vi "Dashboard Main.vi"() -> ()   [LabVIEW 2016]
uses:
  <vilib>/Utility/miscctls.llb/LVRowAndColumnTypeDef.ctl
  <vilib>/event_ctls.llb/eventvkey.ctl
  <vilib>/Rock Robotics/Network Tables/NT Read Boolean.vi
  <vilib>/Rock Robotics/Network Tables/NT Write Boolean.vi
  <vilib>/Rock Robotics/WPI/Dashboard/WPI_DashboardLogging Global.vi
panel:
  in  "Camera Settings Right":T1={"Frame Rate"=30, "Compression"=30, "Size"=1, "DB Camera Config"=FALSE} {"Frame Rate" scale=1.0..30.0; "Compression" scale=100.0..-1.0; "Size" items=["640x480", "320x240", "160x120"]}
  in  "Camera Name Right":string(combo)="No Camera Selection"
  out "Camera Info":cluster{"Mbps LED":bool, "Mbps":dbl, "fps":dbl} {"fps" format="%#.1g"; "Mbps" format="%#.1g"}
  in  "Camera Settings":T1={"Frame Rate"=30, "Compression"=30, "Size"=1, "DB Camera Config"=FALSE} {"Frame Rate" scale=1.0..30.0; "Compression" scale=100.0..-1.0; "Size" items=["640x480", "320x240", "160x120"]}
  in  "TCP":refnum<k5>
  in  "Rec Mode":enum32{"Stop", "Record", "Playback"}(radio)
  out "Robot IP":string
  out "Image Message":string="Timeout in Camera Communications"
  in  "Dashboard Tab":T2(tab)
  in  "Select Auto":string(combo)="Select Autonomous ..."
  out "NT Connection":bool
  out "JS1 Z":dbl(slide) scale=-1.0..1.0 scale format="%#_2e"
  out "JS1 Graph":cluster{"X":dbl, "Y":dbl}[](graph)
  out "JS1 Buttons":T3
  out "JS2 Z":dbl(slide) scale=-1.0..1.0 scale format="%#_2e"
  out "JS2 Graph":cluster{"X":dbl, "Y":dbl}[](graph)
  out "JS2 Buttons":T3
  out "Mode":T4(ring)=enum."Auto Disabled"
  out "Camera Image Right":T5(plugin-control)
  in  "DB/String 9":string
  in  "DB/String 8":string
  in  "DB/String 7":string
  in  "DB/String 6":string
  in  "DB/String 5":string
  in  "DB/String 4":string
  in  "DB/String 3":string
  in  "DB/String 2":string
  in  "DB/String 1":string
  in  "DB/String 0":string
  in  "DB/Slider 0":dbl(slide) scale=0.0..5.0
  in  "DB/Slider 1":dbl(slide) scale=0.0..5.0
  in  "DB/Slider 2":dbl(slide) scale=0.0..5.0
  in  "DB/Slider 3":dbl(slide) scale=0.0..5.0
  out "DB/LED 3":bool
  out "DB/LED 2":bool
  out "DB/LED 1":bool
  out "DB/LED 0":bool
  in  "DB/Button 3":bool
  in  "DB/Button 2":bool
  in  "DB/Button 1":bool
  in  "DB/Button 0":bool caption="New Name"
  in  "Station3":bool
  in  "Station2":bool
  in  "Station1":bool
  in  "ClimberSpeed":dbl(slide)=0.9067796610169492 scale=0.0..1.0
  out "Commanded Angle":dbl
  out "Sonar-Inches":dbl
  out "Encoder-Inches":dbl
  out "Gyro-Degrees":dbl
  out "Battery V":dbl
  out "Doors":bool
  out "Compressor":bool
  in  "Min Area Size %":dbl=20.0
  in  "Lower Threshold":dbl=50.0
  out "Hook Center":dbl
  in  "Test Slider":dbl(slide) scale=0.0..100.0 scale format="%#_3g"
  in  "On/Off":bool caption="Solenoid"
  in  "Test Name":u16(ring) items=["Select the test to run..."]
  in  "Test Tree":string(tree)
  in  "Motor":cluster{"Value":dbl, "Enable":bool} {"Value" scale=-1.0..1.0 scale format="%#_3g"}
  out "Progress":T6 {"Test Progress" scale=0.0..100.0}
  in  "Rev/Fwd":cluster{"Forward":bool, "Reverse":bool}
  in  "Test Ring":u16(ring) items=["Monochrome", "Color"]
  out "Cmd Status":string
  in  "Execute Command":bool
  in  "Command Params":string[][](table)
  in  "Command Selection":i32(listbox)
  in  "CheckList":i32(listbox)
  out "Tree":string(tree)
  out "Camera Image":T5(plugin-control)
  out "Background":bool
  in  "Camera Name":string(combo)="No Camera Selection"
  # "HW"
  # "HW"
  # "Joysticks"
  # "Drive Motors"
  # "Front"
  # "Right"
  # "Left"
  # "Back"
  # "Closed"
  # "Open"
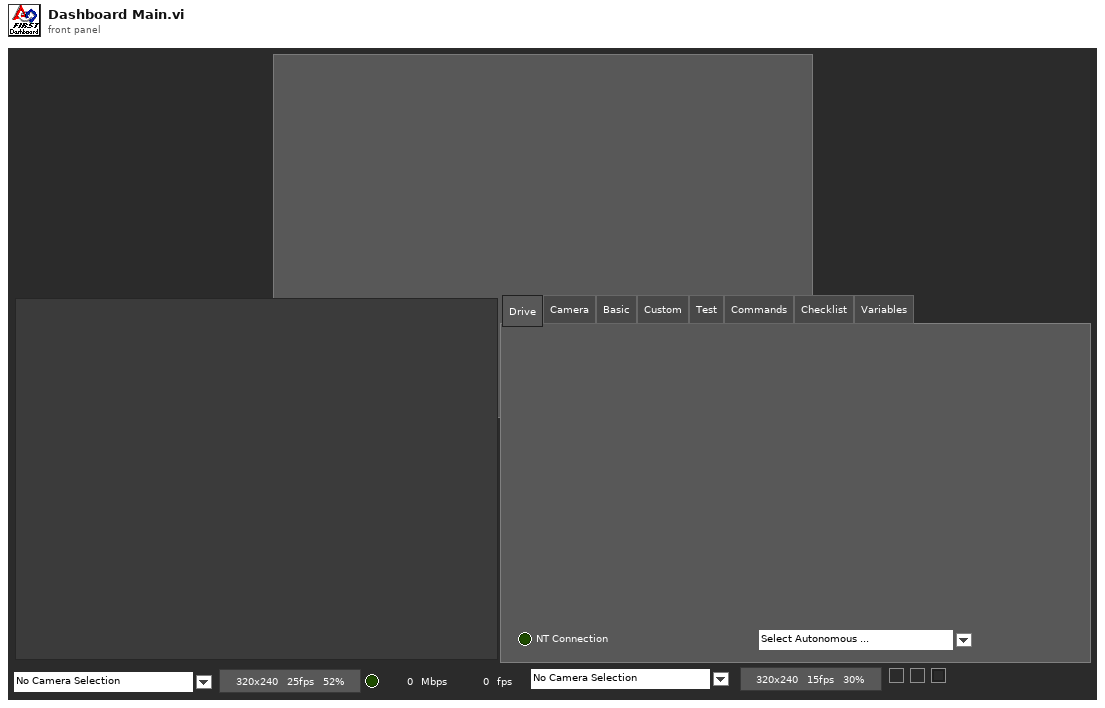
[diagram p1: front panel]
types:
  T1 = cluster{"Frame Rate":i32, "Compression":i32, "Size":u16, "DB Camera Config":bool}
  T2 = enum32{"Drive", "Camera", "Basic", "Custom", "Test", "Commands", "Checklist", "Variables"}
  T3 = cluster{bool, bool, bool, bool, bool, bool, bool, bool, bool, bool, bool, bool}
  T4 = enum8{"Tele-Op Disabled", "Tele-Op Enabled", "Auto Disabled", "Auto Enabled", "Test Disabled", "Test Enabled", "Disconnected", "No Code", "E-Stop"}
  T5 = typedef "IMAQ Image.ctl" = refnum<image>
  T6 = cluster{"Test Progress":u8, "Test Progress Text":string}
  T7 = typedef "Image Type" = u32
  T8 = cluster{"IDs":cluster{"RPC field ID":u16, "Unique ID":u16}, "String":string}
  T9 = enum32{"Drive", "Basic", "Custom", "Test", "Checklist", "Variables"}
  T10 = cluster{"Camera Image":refnum<vi>, "Dashboard Tab":refnum<vi>, "Background":refnum<vi>, "Rec Mode":refnum<vi>, "Test Slider":refnum<vi>, "On/Off ":refnum<vi>, "Test Ring":refnum<vi>, "Rev/Fwd":refnum<vi>, "Test Name":refnum<vi>, "Motor":refnum<vi>, "Progress":refnum<vi>, "CheckList":refnum<vi>, "Tree":refnum<vi>, "Test Tree":refnum<vi>, "Command Params":refnum<vi>, "Command Selection":refnum<vi>, "Execute Command":refnum<vi>, "Cmd Status":refnum<vi>, "Camera Settings":refnum<vi>, "Camera Name":refnum<vi>, "Camera Info":refnum<vi>, "Camera Settings Right":refnum<vi>, "Camera Name Right":refnum<vi>, "Camera Image Right":refnum<vi>}
  T11 = cluster{"Error Strings":string, "Disable Counts":cluster{u16, u16}, "Rail Faults":cluster{u16, u16, u16}, "Robot IP":string, "DB Mode":u8, "Event Info":cluster{"Name":string, "Type":u8, "Number":u16, "Replay":u8}}
  T12 = cluster{"Storage":cluster{"Disk Free":u64, "RAM Block":u32, "RAM free":u32}, "CPU Utilization":cluster{"CPU % ISR":sgl, "CPU % Time Crit":sgl, "CPU % Timed Str":sgl, "CPU % High":sgl, "CPU % Above":sgl, "CPU % Normal":sgl, "CPU % Low":sgl}, "CAN":cluster{"% Bus Utilization":sgl, "Bus Off Cnt":u32, "TX_FIFO Full Cnt":u32, "Receive Error Cnt":u8, "Transmit Error Cnt":u8}, "HID":cluster{"HID Outputs":u32, "Rumble Low":u16, "Rumble High":u16}[]}
  T13 = cluster{"Status bits":cluster{"Test Mode":bool, "Autonomous":bool, "Enabled":bool, "Code Start":bool, "Brownout":bool, "Reserved 2":bool, "Reserved 3":bool, "E-Stop":bool}, "Code Trace":cluster{"Disabled":bool, "TeleOp":bool, "Auto":bool, "Test":bool}, "Controller Type":enum16{"unknown", "cRIO", "roboRio"}, "Code?":enum16{"unknown", "noCode", "code"}, "Battery V":dbl}
  T14 = cluster{"Control Bits":cluster{"TestMode":bool, "Autonomous":bool, "Enabled":bool, "FMS Present":bool, bool, bool, bool, "E-Stop":bool}, "Team Station ":u8, "Countdown":sgl, "Joystick Values":cluster{"Axes":dbl[], "Buttons":bool[], "POVs":i16[]}[]}
  T15 = cluster{"Axes":dbl[], "Buttons":bool[], "POVs":i16[]}[]
  T16 = cluster{"Axes":dbl[], "Buttons":bool[], "POVs":i16[]}
  T17 = cluster{"Buttons[0]":bool, "Buttons[1]":bool, "Buttons[2]":bool, "Buttons[3]":bool, "Buttons[4]":bool, "Buttons[5]":bool, "Buttons[6]":bool, "Buttons[7]":bool, "Buttons[8]":bool, "Buttons[9]":bool, "Buttons[10]":bool, "Buttons[11]":bool}
  T18 = cluster{"Operation":enum16{"Update", "Clear"}, "Color Box":u32}[]
  T19 = typedef "eventvkey.ctl" = enum16{"ASCII", "Enter", "Return", "Shift", "Ctrl", "Alt", "Cmd", "Opt", "Caps", "NumLock", "Clear", "Break", "Up", "Down", "Left", "Right", "Insert", "Delete", "Home", "End", "PageUp", "PageDown", "Escape", "Help", "Pause", "ScrollLock", "F1", "F2", "F3", "F4", "F5", "F6", "F7", "F8", "F9", "F10", "F11", "F12", "F13", "F14", "F15", "F16", "F17", "F18", "F19", "F20", "F21", "F22", "F23", "F24", "Play", "VolumeUp", "VolumeDown", "Mute", "Two Byte Char"}
  T20 = cluster{"Image Size":bool, "Image Type":bool, "Pixel Value":bool, "ROI Information":bool, "Zoom Factor":bool}
  T21 = cluster{"Operation":enum16{"Update", "Clear"}, "Color Box":u32}
  T22 = typedef "LVRowAndColumnTypeDef.ctl" = cluster{"Row":i32, "Column":i32}
  T23 = cluster{"Shift":bool, "Ctrl":bool, "Alt":bool, "Cmd":bool, "Opt":bool}
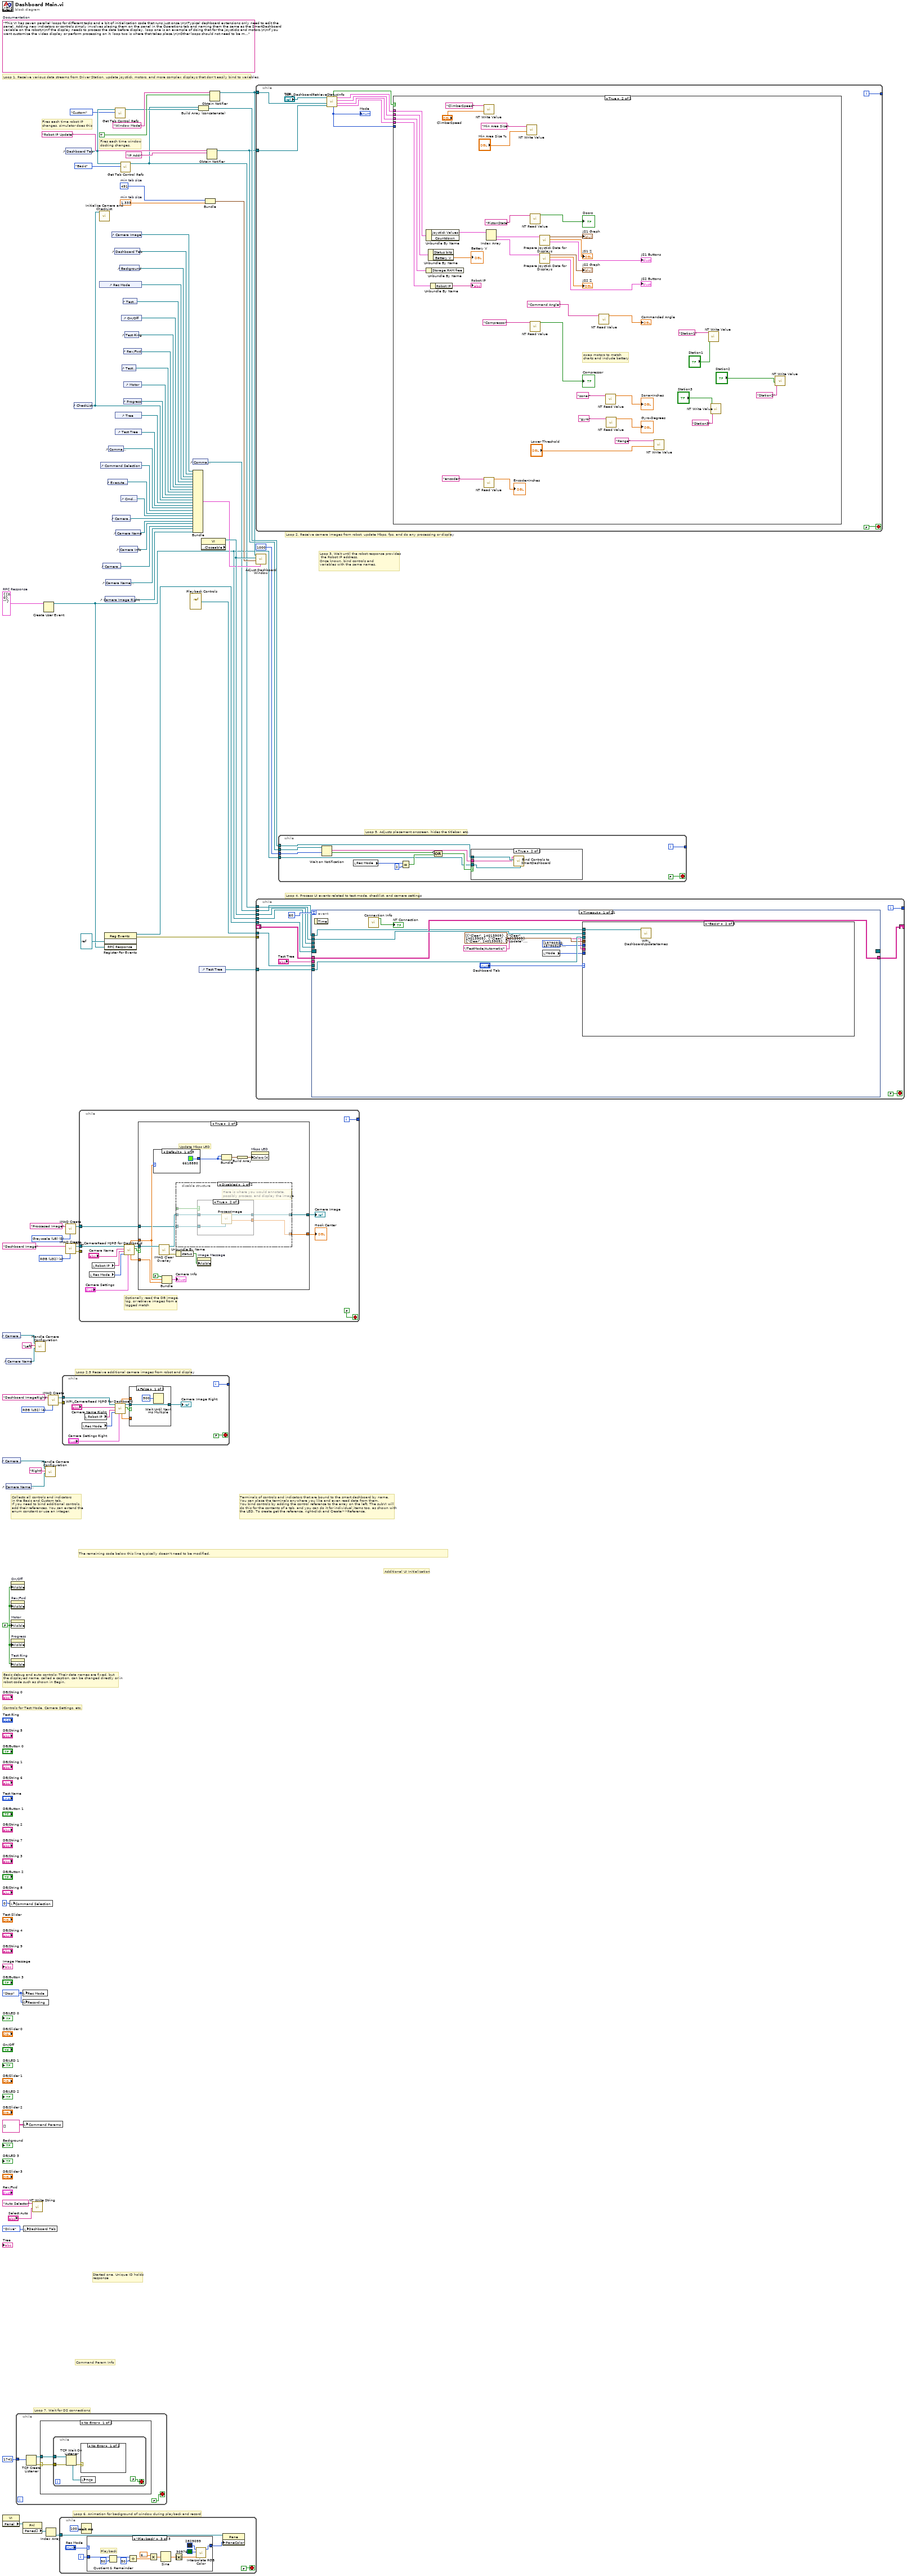
[diagram p0: block diagram]
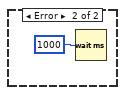
[diagram p3: hidden frame]
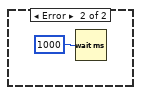
[diagram p4: hidden frame]
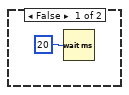
[diagram p5: hidden frame]
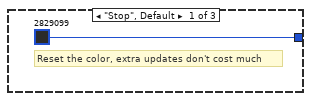
[diagram p6: hidden frame]
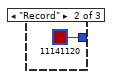
[diagram p7: hidden frame]
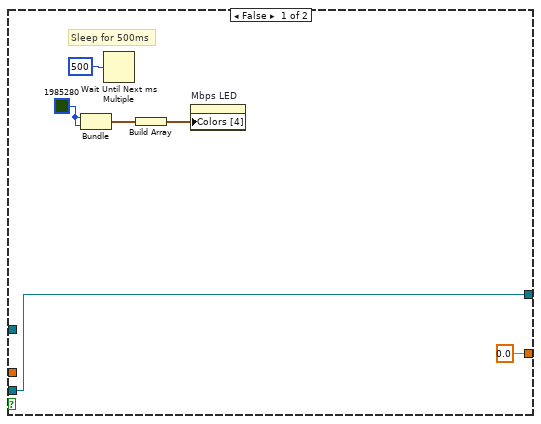
[diagram p9: hidden frame]
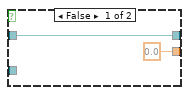
[diagram p10: hidden frame]
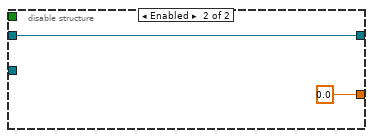
[diagram p11: hidden frame]
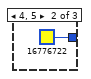
[diagram p12: hidden frame]
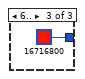
[diagram p13: hidden frame]
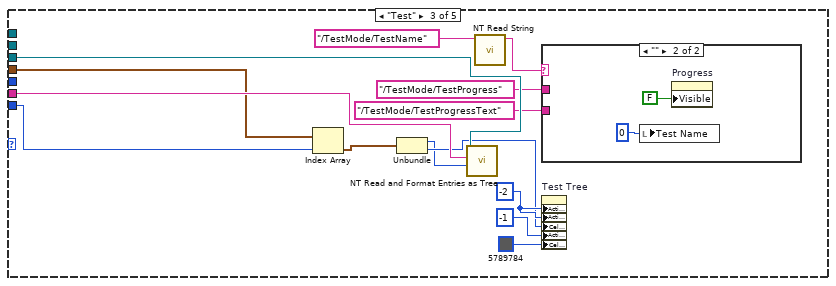
[diagram p15: hidden frame]
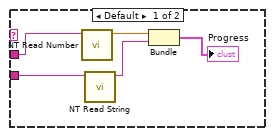
[diagram p16: hidden frame]
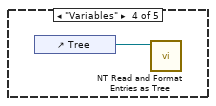
[diagram p17: hidden frame]
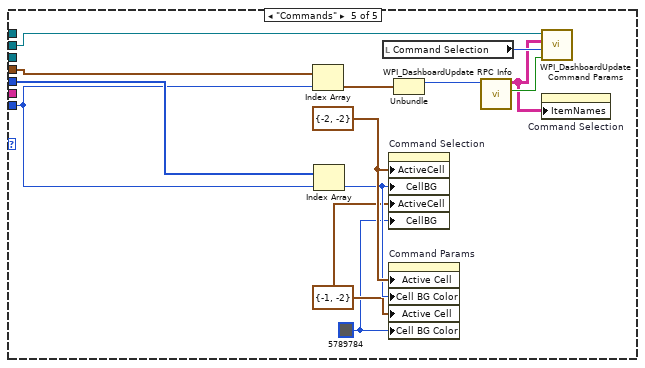
[diagram p18: hidden frame]
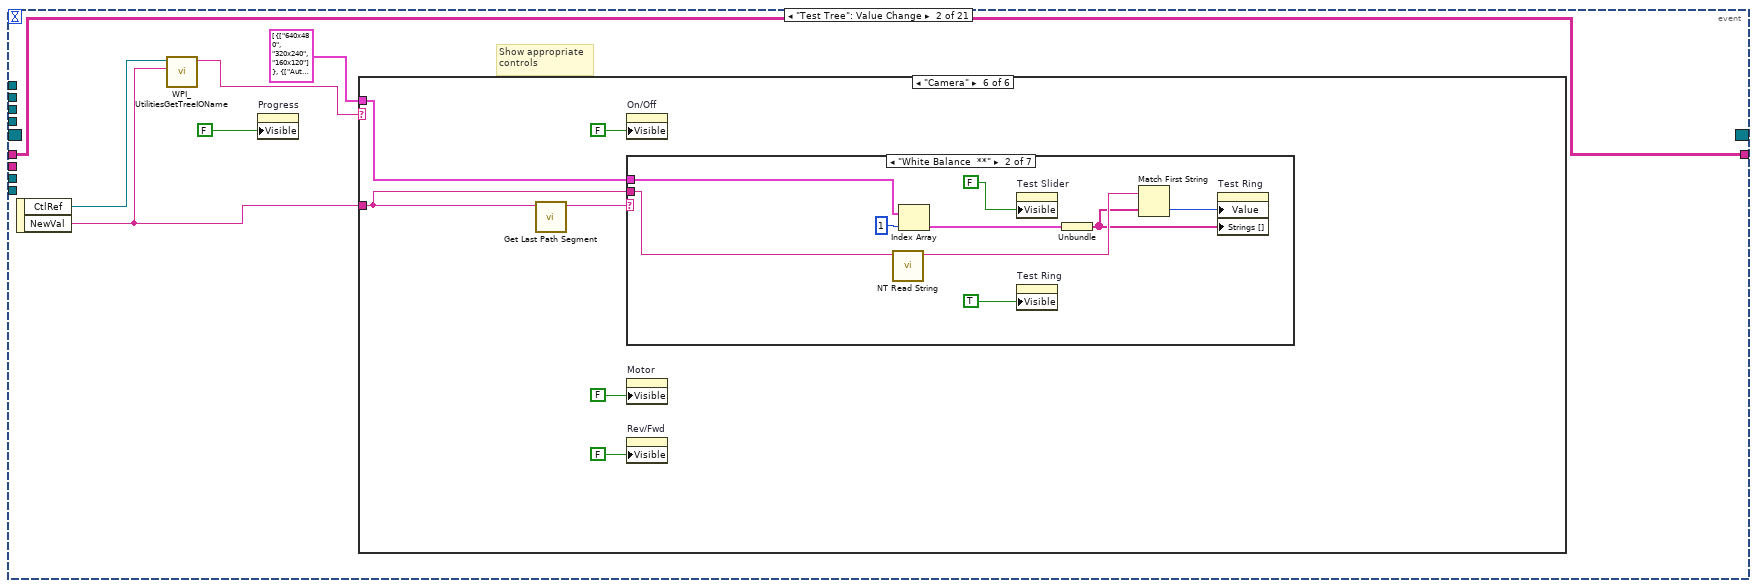
[diagram p19: hidden frame]
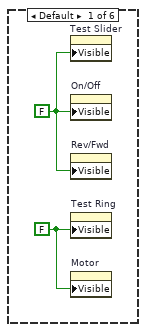
[diagram p20: hidden frame]
diagram:
  w2 = T7 0 items=["Grayscale (U8)", "Grayscale (I16)", "Grayscale (SGL)", "Complex (CSG)", "RGB (U32)", "HSL (U32)", "RGB (U64)"] ("Image Type")
  w13 = T7 4 items=["Grayscale (U8)", "Grayscale (I16)", "Grayscale (SGL)", "Complex (CSG)", "RGB (U32)", "HSL (U32)", "RGB (U64)"] ("Image Type")
  w29 = T8 {"IDs"={"RPC field ID"=0, "Unique ID"=0}, "String"=""}  # RPC Response
  w54 = 491  # min tab size
  w53 = 1.333  # min tab size
  w61 = enum32{"Stop", "Record", "Playback"}."Stop" ("Rec Mode")
  w36 = FALSE ("Visible")
  (unwired) "This VI has seven parallel loops for different tasks and a bit of initialization code that runs just once.\n\nTypical dashboard extensions only need to edit the panel. Adding new indicators or controls simply involves placing them on the panel in the Operations tab and naming them the same as the SmartDashboard variable on the robot\n\nIf the display needs to process the data before display, loop one is an example of doing that for the joysticks and motors.\n\nIf you want customize the video display or perform processing on it, loop two is where that takes place.\n\nOther loops should not need to be modified. They are pretty standard, and document the task they perform."  # Documentation
  w78 = T7 4 items=["Grayscale (U8)", "Grayscale (I16)", "Grayscale (SGL)", "Complex (CSG)", "RGB (U32)", "HSL (U32)", "RGB (U64)"] ("Image Type")
  # "Loop 2.5 Receive additional camera images from robot and display"
  # "Command Param Info"
  # "Started one, Unique ID holds\nresponse"
  # "Loop 7. Wait for DS connections"
  # "Basic debug and auto controls: Their data names are fixed, but\nthe displayed name, called a caption, can be changed directly or in\nrobot code such as shown in Begin."
  # "Controls for Test Mode, Camera Settings, etc."
  # "Additional UI Initialization"
  # "Loop 6. Animation for background of window during playback and record"
  # "Fires each time robot IP\nchanges, simulator does this"
  # "Fires each time window\ndocking changes."
  # "Collects all controls and indicators\nin the Basic and Custom tab.\nIf you need to bind additional controls,\nadd their references. You can extend the\nenum constant or use an integer."
  # "The remaining code below this line typically doesn't need to be modified."
  # "Loop 4. Process UI events related to test mode, checklist, and camera settings"
  # "Terminals of controls and indicators that are bound to the smart dashboard by name.\nYou can place the terminals anywhere you like and even read data from them.\nYou bind controls by adding the control reference to the array on the left. The subVI will\ndo this for the contents of a tab, and you can do it for individual items too, as shown with\nthe LED. To create get the reference, right-click and Create>>Reference."
  # "Loop 3. Wait until the robot response provides\n the Robot IP address.\nOnce known, bind controls and\nvariables with the same names."
  # "Loop 5. Adjusts placement onscreen, hides the titlebar, etc."
  # "Loop 1. Receive various data streams from Driver Station, update joystick, motors, and more complex displays that don't easily bind to variables."
  # "Loop 2. Receive camera images from robot, update Mbps, fps, and do any processing or display"
  n1 = control-ref of="Camera Settings"() -> (w22:refnum<vi>)
  n2 = control-ref of="Camera Settings Right"() -> (w10:refnum<vi>)
  n3 = property class="VI"() -> ("Panel"=w68:refnum<vi>)  [unwired: 2 in, 2 out]
  n4 = control-ref of="Camera Name"() -> (w21:refnum<vi>)
  n5 = control-ref of="Camera Name Right"() -> (w9:refnum<vi>)
  n6 = local write "Command Selection"(u16 0 ("milliseconds to wait")) -> ()
  n7 = property on="On/Off" class="Bool (strict)"("Visible"=w36) -> ()  [unwired: 2 in, 2 out]
  n8 = property on="Rev/Fwd" class="Clust (strict)"("Visible"=w36) -> ()  [unwired: 2 in, 2 out]
  n9 = property on="Motor" class="Clust (strict)"("Visible"=w36) -> ()  [unwired: 2 in, 2 out]
  n10 = property on="Progress" class="Clust (strict)"("Visible"=w36) -> ()  [unwired: 2 in, 2 out]
  n11 = property on="Test Ring" class="Ring (strict)"("Visible"=w36) -> ()  [unwired: 2 in, 2 out]
  n12 = while {
    tunnel: u16 1741 ("timeout ms (25000)") -> [w80]
    stop <- FALSE stop-if-true
    n13 = TCP Create Listener(10:w80) -> (0:w79:errorcluster, 3:w81:refnum<k5>)  [unwired: 4 in, 1 out]
    n14 = case shown="No Error" w79 {
      selector: w79 -> [w83 _]
      tunnel: w81 -> [w84 _]
      frame No Error {
        n15 = while {
          tunnel: w84 -> [w87]
          tunnel: w83 -> [w86]
          stop <- FALSE stop-if-true
          n16 = TCP Wait On Listener(8:w86, 11:w87) -> (0:w88:errorcluster, 4:w89:refnum<k5>)  [unwired: 2 in, 3 out]
          n17 = case shown="No Error" w88 {
            frame No Error {
            }
            frame Error {
              n18 = Wait (ms)(milliseconds to wait=u32 1000) -> ()  [unwired: 1 out]
            }
          }
          n19 = local write "TCP"(w89) -> ()
        }
      }
      frame Error {
        n20 = Wait (ms)(milliseconds to wait=u32 1000) -> ()  [unwired: 1 out]
      }
    }
  }
  n21 = local write "Rec Mode"(w61) -> ()
  n22 = global write "WPI_DashboardLogging Global.vi" "Recording"(w61) -> ()
  n23 = property class="Pnl"(reference=w68) -> ("Panes[]"=w69:refnum<vi>[])  [unwired: 1 in, 2 out]
  n24 = local write "Command Params"(string[][] [] ("Command Params")) -> ()
  n25 = local write "Dashboard Tab"(T2."Drive" ("Dashboard Tab")) -> ()
  n26 = call <vilib>:"NT Write String.vi"("String"="Select Auto", "Name"="Auto Selector") -> ()  [unwired: 9 in, 1 out]
  n27 = call "Handle Camera Configuration.vi"("CameraNameRef"=w21, "Camera File Name"="Left", "ClusterRef"=w22) -> ()  [unwired: 9 in]
  n28 = Create User Event(user event datatype=w29) -> (user event=w25:refnum<user-event>)  [unwired: 1 in, 1 out]
  n29 = call "Handle Camera Configuration.vi"("CameraNameRef"=w9, "Camera File Name"="Right", "ClusterRef"=w10) -> ()  [unwired: 9 in]
  n30 = Index Array(array=w69) -> (element=w67:refnum<vi>)  [unwired: 1 in]
  n31 = call "IMAQ Create"("Image Name"="Dashboard ImageRight", "Image Type"=w13) -> ("New Image"=w12:T5, "error out"=w11:errorcluster)  [unwired: 2 in, 1 out]
  n32 = while {
    tunnel: w67 -> [w93]
    i -> [w96]
    stop <- FALSE stop-if-true
    n33 = Wait (ms)(milliseconds to wait=u32 100) -> ()  [unwired: 1 out]
    n34 = case shown="\"Playback\"" "Rec Mode" {
      tunnel: w96 -> [_ _ w111]
      tunnel: [u32 2829099 ("Base Color") u32 11141120 ("Target Color") w100] -> w92
      frame "Stop", Default {
        # "Reset the color, extra updates don't cost much"
      }
      frame "Record" {
      }
      frame "Playback" {
        # "Playback"
        n35 = Quotient & Remainder(x=w111, y=u32 50 ("milliseconds to wait")) -> (x-y*floor(x/y)=w107:u32)  [unwired: 1 out]
        n36 = Divide(x=w107, y=u32 50 ("milliseconds to wait")) -> (x/y=w104:dbl)
        n37 = Multiply(x=6.283185307179586, y=w104) -> (x*y=w109:dbl)
        n38 = Sine(x=w109) -> (sin(x)=w108:dbl)
        n39 = Absolute Value(x=w108) -> (abs(x)=w101:dbl)
        n40 = call "Interpolate RGB Color.vi"("Proportion"=w101, "Target Color"=u32 30976, "Base Color"=u32 2829099) -> ("Result Color"=w100:u32)  [unwired: 8 in]
      }
    }
    n41 = property class="Pane"(reference=w93, "PaneColor"=w92) -> ()  [unwired: 1 in, 2 out]
  }
  n42 = while {
    tunnel: w12 -> [w122]
    tunnel: w11 -> [_]
    tunnel: [w116] -> _
    i -> [w116]
    stop <- FALSE stop-if-true
    n43 = local read "Rec Mode"() -> (w120:enum32{"Stop", "Record", "Playback"})
    n44 = local read "Robot IP"() -> (w121:string)
    n45 = call <vilib>:"WPI_CameraRead MJPG for Dashboard.vi"("Camera Settings"="Camera Settings Right", "Rec Mode"=w120, "Robot IP"=w121, "Camera Name"="Camera Name Right", "Refnum in"=w122) -> ("Active"=w115:bool, "Refnum out"=w118:T5, "FPS"=w113:dbl, "Bandwidth (Mbps)"=w114:dbl)  [unwired: 3 in]
    n46 = case shown="False" w115 {
      tunnel: w118 -> [w124 w126]
      tunnel: w114 -> [_ _]
      tunnel: w113 -> [_ _]
      tunnel: [w124 w126] -> w112
      frame False {
        n47 = Wait Until Next ms Multiple(millisecond multiple=u32 500) -> ()  [unwired: 1 out]
      }
      frame True {
      }
    }
    "Camera Image Right" <- w112
  }
  n48 = control-ref of="Dashboard Tab"() -> (w59:refnum<vi>)
  n49 = call "IMAQ Create"("Image Name"="Proccesed Image", "Image Type"=w2) -> ("New Image"=w1:T5)  [unwired: 2 in, 2 out]
  n50 = call "IMAQ Create"("Image Name"="Dashboard Image", "Image Type"=w78) -> ("New Image"=w76:T5, "error out"=w75:errorcluster)  [unwired: 2 in, 1 out]
  n51 = control-ref of="CheckList"() -> (w47:refnum<vi>)
  n52 = while {
    tunnel: w76 -> [w138]
    tunnel: w75 -> [_]
    tunnel: [w139] -> _
    tunnel: w1 -> [w127]
    i -> [w139]
    stop <- FALSE stop-if-true
    # "Optionally read the DB image,\nlog, or retrieve images from a\nlogged match"
    n53 = local read "Rec Mode"() -> (w134:enum32{"Stop", "Record", "Playback"})
    n54 = local read "Robot IP"() -> (w133:string)
    n55 = call <vilib>:"WPI_CameraRead MJPG for Dashboard.vi"("Camera Settings"="Camera Settings", "Rec Mode"=w134, "Robot IP"=w133, "Camera Name"="Camera Name", "Refnum in"=w138) -> ("Active"=w136:bool, "Refnum out"=w137:T5, "FPS"=w135:dbl, "Bandwidth (Mbps)"=w132:dbl)  [unwired: 3 in]
    n56 = case shown="True" w136 {
      tunnel: w137 -> [w142 w156]
      tunnel: w132 -> [_ w153]
      tunnel: w135 -> [_ w154]
      tunnel: [w142 w148] -> w129
      tunnel: [0.0 ("Numeric") w150] -> w128
      tunnel: w127 -> [_ w147]
      frame False {
        w144 = u32 1985280 ("Color Box")
        # "Sleep for 500ms"
        n57 = Bundle("Color Box"=w144, "Color Box"=w144) -> (w145:cluster{"Color Box":u32, "Color Box":u32})  [unwired: 1 out]
        n58 = Wait Until Next ms Multiple(millisecond multiple=u32 500) -> ()  [unwired: 1 out]
        n59 = Build Array(w145) -> (w143:cluster{"Color Box":u32, "Color Box":u32}[])
        n60 = property on="Mbps LED" class="Bool (strict)"("Colors [4]"=w143) -> ()  [unwired: 2 in, 2 out]
      }
      frame True {
        # "Update Mbps LED"
        n61 = case shown="Default" w153 {
          tunnel: [u32 6618880 ("Color Box") u32 16776722 ("Color Box") u32 16716800 ("Color Box")] -> w157
          frame Default {
          }
          frame 4, 5 {
          }
          frame 6.. {
          }
        }
        n62 = call "IMAQ Clear Overlay"("Image"=w156) -> ("error out"=w159:errorcluster, "Image Out"=w149:T5)  [unwired: 2 in, 7 out]
        n63 = Bundle(FALSE, "Bandwidth (Mbps)"=w153, "FPS"=w154) -> (→"Camera Info":cluster{bool, "Bandwidth (Mbps)":dbl, "FPS":dbl})  [unwired: 1 in]
        n64 = disable-structure shown="Disabled" {
          disable-tunnel: [w165 0.0 ("Numeric")] -> w150
          disable-tunnel: w149 -> [w164 w173]
          disable-tunnel: [w163 w173] -> w148
          disable-tunnel: _ -> [w162 _]
          disable-tunnel: w147 -> [w161 _]
          frame Disabled {
            # "Here is where you would annotate,\npossibly process, and display the image"
            n65 = case shown="True" w162 {
              tunnel: [0.0 ("Numeric") w171] -> w165
              tunnel: w164 -> [w167 w170]
              tunnel: [w167 w169] -> w163
              tunnel: w161 -> [_ w168]
              frame False {
              }
              frame True {
                n66 = call "ProcessImage.vi"("New Image"=w168, "Refnum in"=w170) -> ("Numeric"=w171:dbl, "Refnum out"=w169:T5)  [unwired: 7 in, 1 out]
              }
            }
          }
          frame Enabled {
          }
        }
        n67 = Unbundle By Name(w159) -> ("status"=w160:bool)
        n68 = property on="Image Message" class="Str"("Visible"=w160) -> ()  [unwired: 2 in, 2 out]
        n69 = Bundle("Color Box"=w157, "Color Box"=w157) -> (w158:cluster{"Color Box":u32, "Color Box":u32})  [unwired: 1 out]
        n70 = Build Array(w158) -> (w155:cluster{"Color Box":u32, "Color Box":u32}[])
        n71 = property on="Mbps LED" class="Bool (strict)"("Colors [4]"=w155) -> ()  [unwired: 2 in, 2 out]
      }
    }
    "Camera Image" <- w129
    "Hook Center" <- w128
  }
  n72 = call "Initialize Camera and CheckList.vi"("ListBox in"=w47) -> ()  [unwired: 11 in]
  n73 = control-ref of="Rec Mode"() -> (w42:refnum<vi>)
  n74 = control-ref of="Command Selection"() -> (w28:refnum<vi>)
  n75 = control-ref of="Camera Settings Right"() -> (w6:refnum<vi>)
  n76 = register-events(refnum<vi> refnum, w25) -> (reference out=w65:refnum<event-registration>, error out=w64:errorcluster)  [unwired: 2 in]
  n77 = control-ref of="Camera Image Right"() -> (w4:refnum<vi>)
  n78 = control-ref of="Camera Name Right"() -> (w5:refnum<vi>)
  n79 = control-ref of="Execute Command"() -> (w30:refnum<vi>)
  n80 = control-ref of="Command Params"() -> (w31:refnum<vi>)
  n81 = control-ref of="Camera Image"() -> (w56:refnum<vi>)
  n82 = control-ref of="Camera Settings"() -> (w20:refnum<vi>)
  n83 = control-ref of="Dashboard Tab"() -> (w55:refnum<vi>)
  n84 = control-ref of="Tree"() -> (w46:refnum<vi>)
  n85 = control-ref of="Test Tree"() -> (w45:refnum<vi>)
  n86 = call <vilib>:"Get Tab Control Refs.vi"("Page Index"=T9."Custom" ("Dashboard Tab"), "TabControl in"=w59) -> ("ControlsOnPage"=w58:refnum<vi>[])  [unwired: 9 in]
  n87 = control-ref of="Camera Name"() -> (w19:refnum<vi>)
  n88 = control-ref of="Background"() -> (w51:refnum<vi>)
  n89 = control-ref of="Camera Info"() -> (w18:refnum<vi>)
  n90 = call <vilib>:"Get Tab Control Refs.vi"("Page Index"=T9."Basic" ("Dashboard Tab"), "TabControl in"=w59) -> ("ControlsOnPage"=w17:refnum<vi>[])  [unwired: 9 in]
  n91 = control-ref of="Cmd Status"() -> (w24:refnum<vi>)
  n92 = control-ref of="On/Off"() -> (w40:refnum<vi>)
  n93 = control-ref of="Test Name"() -> (w44:refnum<vi>)
  n94 = control-ref of="Test Slider"() -> (w41:refnum<vi>)
  n95 = control-ref of="Rev/Fwd"() -> (w38:refnum<vi>)
  n96 = control-ref of="Motor"() -> (w43:refnum<vi>)
  n97 = control-ref of="Progress"() -> (w37:refnum<vi>)
  n98 = control-ref of="Test Ring"() -> (w39:refnum<vi>)
  n99 = vi-ref "Playback Controls.vi"() -> (w66:refnum<vi>)
  n100 = control-ref of="Command Params"() -> (w23:refnum<vi>)
  n101 = Bundle("Camera Image"=w56, "Dashboard Tab"=w55, "Background"=w51, "Rec Mode"=w42, "Test Slider"=w41, "On/Off"=w40, "Test Ring"=w39, "Rev/Fwd"=w38, "Test Name"=w44, "Motor"=w43, "Progress"=w37, "CheckList"=w47, "Tree"=w46, "Test Tree"=w45, "Command Params"=w31, "Command Selection"=w28, "Execute Command"=w30, "Cmd Status"=w24, "Camera Settings"=w20, "Camera Name"=w19, "Camera Info"=w18, "Camera Settings Right"=w6, "Camera Name Right"=w5, "Camera Image Right"=w4) -> (w48:T10)  [unwired: 1 in]
  n102 = Build Array (concatenate)(w17, w58) -> (w57:refnum<vi>[])
  n103 = control-ref of="Test Tree"() -> (w70:refnum<vi>)
  n104 = property class="VI" props=["Front Panel.Closeable"]() -> (reference out=w60:refnum<vi>)  [unwired: 2 in, 2 out]
  n105 = Bundle("min tab size"=w54, "min tab size"=w53) -> (w52:cluster{"min tab size":i32, "min tab size":dbl})  [unwired: 1 in]
  n106 = Obtain Notifier(name (unnamed)="Robot IP Update", notification data type="IP Addr" ("name (unnamed)")) -> (notifier out=w35:refnum<notifier>)  [unwired: 2 in, 2 out]
  n107 = Obtain Notifier(name (unnamed)="Window Mode", notification data type=TRUE) -> (notifier out=w34:refnum<notifier>)  [unwired: 2 in, 2 out]
  n108 = while {
    tunnel: [w186] -> _
    tunnel: w35 -> [w180]
    tunnel: w34 -> [w177]
    i -> [w186]
    stop <- FALSE stop-if-true
    n109 = call <vilib>:"WPI_DashboardRetrieveStatusInfo.vi"("Binding Refnum"=w180, "Window Mode Notifier"=w177, "TCP Cnx"="TCP") -> ("Power and Errors"=w181:T11, "Robot Metrics"=w184:T12, "Status Info"=w185:T13, "Control Info"=w182:T14, "Robot Mode"=w179:T4, "Process?"=w183:bool)  [unwired: 3 in]
    "Mode" <- w179
    n110 = case shown="True" w183 {
      tunnel: w185 -> [_ w227]
      tunnel: w184 -> [_ w226]
      tunnel: w182 -> [_ w225]
      tunnel: w181 -> [_ w224]
      tunnel: w179 -> [_ _]
      frame False {
        n111 = Wait (ms)(milliseconds to wait=u32 20) -> ()  [unwired: 1 out]
      }
      frame True {
        # "swap motors to match\ncharts and include battery"
        n112 = Unbundle By Name(w225) -> ("Joystick Values"=w223:T15)  [unwired: 1 out]
        n113 = Unbundle By Name(w226) -> ()  [unwired: 1 out]
        n114 = Unbundle By Name(w227) -> ("Battery V"=→"Battery V":dbl)  [unwired: 1 out]
        n115 = Unbundle By Name(w224) -> ("Robot IP"=→"Robot IP":string)
        n116 = call-poly <vilib>:"NT Write Value.vi"("Numeric"="ClimberSpeed", "Name"="ClimberSpeed") -> ()  [unwired: 9 in, 1 out]
        n117 = call-poly <vilib>:"NT Read Value.vi"("Name"="encoder") -> ("Numeric"=→"Encoder-Inches":dbl)  [unwired: 9 in, 1 out]
        n118 = Index Array(array=w223) -> (element #1=w222:T16, element #2=w218:T16)  [unwired: 2 in]
        n119 = call-poly <vilib>:"NT Write Value.vi"("Numeric"="Min Area Size %", "Name"="Min Area Size") -> ()  [unwired: 9 in, 1 out]
        n120 = call-poly <vilib>:"NT Read Value.vi"("Name"="PistonState") -> ("Boolean"=→"Doors":bool)  [unwired: 9 in, 1 out]
        n121 = call-poly <vilib>:"NT Read Value.vi"("Name"="Compressor") -> ("Boolean"=→"Compressor":bool)  [unwired: 9 in, 1 out]
        n122 = call "Prepare Joystick Data for Displays.vi"("Joystick Values"=w222) -> ("Buttons"=→"JS1 Buttons":T17, "Z Axis"=→"JS1 Z":dbl, "Cartesian Data"=→"JS1 Graph":cluster{"X axis":dbl, "X axis":dbl}[])  [unwired: 8 in]
        n123 = call "Prepare Joystick Data for Displays.vi"("Joystick Values"=w218) -> ("Buttons"=→"JS2 Buttons":T17, "Z Axis"=→"JS2 Z":dbl, "Cartesian Data"=→"JS2 Graph":cluster{"X axis":dbl, "X axis":dbl}[])  [unwired: 8 in]
        n124 = call-poly <vilib>:"NT Read Value.vi"("Name"="Command Angle") -> ("Numeric"=→"Commanded Angle":dbl)  [unwired: 9 in, 1 out]
        n125 = call-poly <vilib>:"NT Read Value.vi"("Name"="sonar") -> ("Numeric"=→"Sonar-Inches":dbl)  [unwired: 9 in, 1 out]
        n126 = call-poly <vilib>:"NT Read Value.vi"("Name"="gyro") -> ("Numeric"=→"Gyro-Degrees":dbl)  [unwired: 9 in, 1 out]
        n127 = call-poly <vilib>:"NT Write Value.vi"("Numeric"="Lower Threshold", "Name"="Range") -> ()  [unwired: 9 in, 1 out]
        n128 = call-poly <vilib>:"NT Write Value.vi"("Boolean"="Station1", "Name"="Station1") -> ()  [unwired: 9 in, 1 out]
        n129 = call-poly <vilib>:"NT Write Value.vi"("Boolean"="Station3", "Name"="Station3") -> ()  [unwired: 9 in, 1 out]
        n130 = call-poly <vilib>:"NT Write Value.vi"("Boolean"="Station2", "Name"="Station2") -> ()  [unwired: 9 in, 1 out]
      }
    }
  }
  n131 = call "Adjust Dashboard Window.vi"("Sizing Refnums"=w48, "Size Constraints"=w52, "VI"=w60, "WIn Mode"=w34) -> ()  [unwired: 8 in]
  n132 = while {
    tunnel: [w237] -> _
    tunnel: w70 -> [w236]
    tunnel: w66 -> [w235]
    tunnel: w65 -> [w234]
    tunnel: w64 -> [_]
    tunnel: w60 -> [w233]
    tunnel: w25 -> [w232]
    tunnel: w23 -> [w231]
    shift-right: [w230] -> _
    shift-left: _ -> [w229]
    tunnel: w17 -> [w228]
    i -> [w237]
    stop <- FALSE stop-if-true
    n133 = event shown="[0] Timeout" {
      selector: w234 -> [_ _ _ _ _ _ _ _ _ _ _ _ _ _ _ _ _ _ _ _ _]
      dyn-events: [_ _ _ _ _ _ _ _ _ _ _ _ _ _ _ _ w493 _ _ _ _] -> _
      timeout: u32 60 ("milliseconds to wait") -> [_ _ _ _ _ _ _ _ _ _ _ _ _ _ _ _ _ _ _ _ _]
      tunnel: w236 -> [w249 _ _ _ _ _ _ _ _ _ _ _ _ _ _ _ _ _ _ _ _]
      tunnel: "Test Tree" -> [_ _ _ _ _ _ _ _ _ _ _ w460 w468 w470 w474 w482 _ _ _ _ _]
      tunnel: w235 -> [_ _ _ _ _ _ _ _ _ _ _ _ _ _ _ _ w495 _ w513 _ _]
      tunnel: w233 -> [_ _ _ _ _ _ _ _ _ _ _ _ _ _ _ _ w491 _ _ _ _]
      tunnel: w232 -> [_ _ _ _ _ _ _ _ _ _ _ _ _ _ _ _ w487 _ _ _ _]
      tunnel: w231 -> [w244 _ _ _ _ _ w411 _ _ _ _ _ _ _ _ _ _ _ _ _ _]
      tunnel: [w243 w288 w390 w395 w404 w408 w409 w418 w428 w435 w447 w459 w466 w469 w473 w481 w486 w508 w510 w514 w525] -> w230
      tunnel: w229 -> [w243 w288 w390 w395 w404 w408 w409 _ _ w435 w447 w459 w466 w469 w473 w481 w486 w508 w510 w514 w525]
      tunnel: w228 -> [w241 _ _ _ _ _ _ _ _ _ _ _ _ _ _ _ _ _ _ _ _]
      event Timeout {
        n134 = event-data() -> ()  [unwired: 1 in, 1 out]
        n135 = call <vilib>:"Connextion Info.vi"() -> ("Connected"=→"NT Connection":bool)  [unwired: 10 in, 1 out]
        n136 = local read "Mode"() -> (w246:T4)
        n137 = case shown="\"Basic\"" "Dashboard Tab" {
          tunnel: w249 -> [_ _ w265 _ _]
          tunnel: "/TestMode/Automatic/" ("Name Pattern") -> [_ _ w264 _ _]
          tunnel: T18 [{"Operation"=enum."Clear", "Color Box"=14013909}, {"Operation"=enum."Clear", "Color Box"=14013909}, {"Operation"=enum."Clear", "Color Box"=14013909}, {"Operation"=enum."Clear", "Color Box"=14013909}, {"Operation"=enum."Update", "Color Box"=14013909}, {"Operation"=enum."Update", "Color Box"=16777215}, {"Operation"=enum."Clear", "Color Box"=14013909}, {"Operation"=enum."Clear", "Color Box"=14013909}, {"Operation"=enum."Clear", "Color Box"=14013909}] -> [_ _ w257 _ w281]
          tunnel: w246 -> [_ _ w256 _ w280]
          tunnel: u32[] [15790320, 15790320, 15790320, 15790320, 16777215, 16777215, 15790320, 15790320, 15790320] -> [_ _ _ _ w286]
          tunnel: w244 -> [_ _ _ _ w274]
          tunnel: w241 -> [_ w251 _ _ _]
          frame "Custom", Default {
          }
          frame "Basic" {
            n138 = call <vilib>:"WPI_DashboardUpdateNames.vi"("Controls on Tab"=w251) -> ()  [unwired: 11 in]
          }
          frame "Test" {
            w263 = -2 ("Active Item:Row Number")
            n139 = Index Array(array=w257, index=w256) -> (element=w258:T21)
            n140 = Unbundle(w258) -> ("Operation"=w259:enum16{"Update", "Clear"}, "Color Box"=w260:u32)
            n141 = call <vilib>:"NT Read and Format Entries as Tree.vi"("Operation"=w259, "Name Pattern"=w264, "Tree Refnum"=w265) -> ()  [unwired: 7 in, 2 out]
            n142 = call <vilib>:"NT Read String.vi"("Name"="/TestMode/TestName") -> ("String"=w254:string)  [unwired: 9 in, 1 out]
            n143 = case shown="\"\"" w254 {
              tunnel: "/TestMode/TestProgress" ("Name") -> [w267 _]
              tunnel: "/TestMode/TestProgressText" ("Name") -> [w266 _]
              frame Default {
                n144 = call <vilib>:"NT Read Number.vi"("Name"=w267) -> ("Numeric"=w268:dbl)  [unwired: 9 in, 1 out]
                n145 = call <vilib>:"NT Read String.vi"("Name"=w266) -> ("String"=w269:string)  [unwired: 9 in, 1 out]
                n146 = Bundle("Numeric"=w268, "String"=w269) -> (→"Progress":cluster{"Numeric":dbl, "String":string})  [unwired: 1 in]
              }
              frame "" {
                n147 = local write "Test Name"(u16 0) -> ()
                n148 = property on="Progress" class="Clust (strict)"("Visible"=FALSE) -> ()  [unwired: 2 in, 2 out]
              }
            }
            n149 = property on="Test Tree" class="Tree (strict)"("Active Item Row Number"=w263, "ActiveColNum"=w263, "CellBG"=w260, "Active Item Row Number"=-1 ("Active Item:Row Number"), "CellBG"=u32 5789784 ("Color Box")) -> ()  [unwired: 2 in, 2 out]
          }
          frame "Variables" {
            n150 = control-ref of="Tree"() -> (w273:refnum<vi>)
            n151 = call <vilib>:"NT Read and Format Entries as Tree.vi"("Tree Refnum"=w273) -> ()  [unwired: 9 in, 2 out]
          }
          frame "Commands" {
            w282 = u32 5789784 ("Color Box")
            w283 = T22 {"Row"=-1, "Column"=-2} ("Active Cell:Active Cell")
            w285 = T22 {"Row"=-2, "Column"=-2} ("Active Cell:Active Cell")
            n152 = Index Array(array=w281, index=w280) -> (element=w279:T21)
            n153 = Index Array(array=w286, index=w280) -> (element=w284:u32)
            n154 = local read "Command Selection"() -> (w277:i32)
            n155 = property on="Command Selection" class="MCListbox (strict)"("ActiveCell"=w285, "CellBG"=w284, "ActiveCell"=w283, "CellBG"=w282) -> ()  [unwired: 2 in, 2 out]
            n156 = property on="Command Params" class="Tbl (strict)"("Active Cell"=w285, "Cell BG Color"=w284, "Active Cell"=w283, "Cell BG Color"=w282) -> ()  [unwired: 2 in, 2 out]
            n157 = Unbundle(w279) -> ("Operation"=w278:enum16{"Update", "Clear"})  [unwired: 1 out]
            n158 = call <vilib>:"WPI_DashboardUpdate RPC Info.vi"("Operation"=w278) -> ("update"=w276:bool, "commands"=w275:string[][])  [unwired: 9 in]
            n159 = call <vilib>:"WPI_DashboardUpdate Command Params.vi"("Update"=w276, "NewVal"=w277, "Commands"=w275, "Param Tbl"=w274) -> ()  [unwired: 7 in, 1 out]
            n160 = property on="Command Selection" class="MCListbox (strict)"("ItemNames"=w275) -> ()  [unwired: 2 in, 2 out]
          }
        }
      }
      event "Test Tree": Value Change {
        # "Show appropriate\ncontrols"
        n161 = event-data() -> ("CtlRef"=w291:refnum<vi>, "NewVal"=w289:string)  [unwired: 1 in]
        n162 = call <vilib>:"WPI_UtilitiesGetTreeIOName.vi"("NewVal"=w289, "TreeControl in"=w291) -> ("I/O Name"=w292:string)  [unwired: 9 in]
        n163 = property on="Progress" class="Clust (strict)"("Visible"=FALSE) -> ()  [unwired: 2 in, 2 out]
        n164 = case shown="\"Camera\"" w292 {
          selector: w292 -> [_ w299 _ w321 w330 _]
          tunnel: w289 -> [_ _ w318 w320 _ w337]
          tunnel: cluster{string[]}[] [{["640x480", "320x240", "160x120"]}, {["Auto", "Fixed indoor", "Fixed outdoor 1", "Fixed outdoor 2", "Fixed fluorescent 1", "Fixed fluorescent 2", "Hold current"]}, {["Auto", "Flicker-free 50 Hz", "Flicker-free 60 Hz", "Hold current"]}, {["None", "Prioritize frame rate", "Prioritize image quality"]}, {["Monochrome", "Color"]}] -> [_ _ _ _ _ w336]
          frame Default {
            w294 = FALSE ("Visible")
            w293 = FALSE ("Visible")
            n165 = property on="Test Slider" class="Slide (strict)"("Visible"=w294) -> ()  [unwired: 2 in, 2 out]
            n166 = property on="On/Off" class="Bool (strict)"("Visible"=w294) -> ()  [unwired: 2 in, 2 out]
            n167 = property on="Rev/Fwd" class="Clust (strict)"("Visible"=w294) -> ()  [unwired: 2 in, 2 out]
            n168 = property on="Test Ring" class="Ring (strict)"("Visible"=w293) -> ()  [unwired: 2 in, 2 out]
            n169 = property on="Motor" class="Clust (strict)"("Visible"=w293) -> ()  [unwired: 2 in, 2 out]
          }
          frame "Analog Out", "Motor", "PWM" {
            w300 = FALSE ("Visible")
            n170 = case shown="\"Analog Out\"" w299 {
              tunnel: [1.0 ("Value") -1.0 ("Value") 0.0 ("Value")] -> w298
              tunnel: [255.0 ("Value") 1.0 ("Value") 5.0 ("Value")] -> w297
              tunnel: [128.0 ("Value") 0.0 ("Value") 0.0 ("Value")] -> w296
              tunnel: [64.0 ("Value") 0.5 ("Value") 1.0 ("Value")] -> w295
              frame "PWM" {
              }
              frame "Motor", Default {
              }
              frame "Analog Out" {
              }
            }
            n171 = property on="Test Slider" class="Slide (strict)"("Visible"=w300) -> ()  [unwired: 2 in, 2 out]
            n172 = property on="Test Ring" class="Ring (strict)"("Visible"=w300) -> ()  [unwired: 2 in, 2 out]
            n173 = property on="On/Off" class="Bool (strict)"("Visible"=w300) -> ()  [unwired: 2 in, 2 out]
            n174 = property on="Rev/Fwd" class="Clust (strict)"("Visible"=w300) -> ()  [unwired: 2 in, 2 out]
            n175 = property on="Motor" class="Clust (strict)"("Visible"=TRUE) -> ()  [unwired: 2 in, 2 out]
            n176 = property on="Value" class="Slide (strict)"("Value"=w296, "Scale.Minimum"=w298, "Scale.Maximum"=w297, "Scale.Increment"=w295) -> ()  [unwired: 2 in, 2 out]
          }
          frame "Servo" {
            w316 = FALSE ("Visible")
            n177 = call <vilib>:"NT Read Number.vi"("Name"=w318) -> ("Numeric"=w317:dbl)  [unwired: 9 in, 1 out]
            n178 = property on="Motor" class="Clust (strict)"("Visible"=w316) -> ()  [unwired: 2 in, 2 out]
            n179 = property on="Test Ring" class="Ring (strict)"("Visible"=w316) -> ()  [unwired: 2 in, 2 out]
            n180 = property on="On/Off" class="Bool (strict)"("Visible"=w316) -> ()  [unwired: 2 in, 2 out]
            n181 = property on="Rev/Fwd" class="Clust (strict)"("Visible"=w316) -> ()  [unwired: 2 in, 2 out]
            n182 = property on="Test Slider" class="Slide (strict)"("Visible"=TRUE, "Scale.Maximum"=170.0 ("Scale.Range:Maximum")) -> ()  [unwired: 2 in, 2 out]
            n183 = local write "Test Slider"(w317) -> ()
          }
          frame "Relay", "Solenoid" {
            w319 = FALSE ("Visible")
            n184 = property on="Motor" class="Clust (strict)"("Visible"=w319) -> ()  [unwired: 2 in, 2 out]
            n185 = property on="Test Slider" class="Slide (strict)"("Visible"=w319) -> ()  [unwired: 2 in, 2 out]
            n186 = property on="Test Ring" class="Ring (strict)"("Visible"=w319) -> ()  [unwired: 2 in, 2 out]
            n187 = Search and Replace String(input string=w320, search string="/Value  **", replace string="/Direction") -> (result string=w326:string)  [unwired: 5 in, 3 out]
            n188 = call <vilib>:"NT Read String.vi"("Name"=w326) -> ("String"=w324:string)  [unwired: 9 in, 1 out]
            n189 = Equal?(x="Both directions", y=w324) -> (x = y?=w322:bool)
            n190 = property on="Rev/Fwd" class="Clust (strict)"("Visible"=w322) -> ()  [unwired: 2 in, 2 out]
            n191 = Not(x=w322) -> (.not. x?=w323:bool)
            n192 = property on="On/Off" class="Bool (strict)"("Visible"=w323, "Caption.Text"=w321) -> ()  [unwired: 2 in, 2 out]
          }
          frame "Compressor", "Digital Out" {
            w329 = FALSE ("Visible")
            # "Get direction and finish"
            n193 = property on="Rev/Fwd" class="Clust (strict)"("Visible"=FALSE) -> ()  [unwired: 2 in, 2 out]
            n194 = property on="Test Ring" class="Ring (strict)"("Visible"=w329) -> ()  [unwired: 2 in, 2 out]
            n195 = property on="Motor" class="Clust (strict)"("Visible"=w329) -> ()  [unwired: 2 in, 2 out]
            n196 = property on="Test Slider" class="Slide (strict)"("Visible"=w329) -> ()  [unwired: 2 in, 2 out]
            n197 = property on="On/Off" class="Bool (strict)"("Visible"=TRUE, "Caption.Text"=w330) -> ()  [unwired: 2 in, 2 out]
          }
          frame "Camera" {
            n198 = call <vilib>:"Get Last Path Segment.vi"("String in"=w337) -> ("String out"=w338:string)  [unwired: 10 in]
            n199 = property on="On/Off" class="Bool (strict)"("Visible"=FALSE) -> ()  [unwired: 2 in, 2 out]
            n200 = case shown="\"White Balance  **\"" w338 {
              tunnel: w337 -> [w344 w353 w362 w371 w380 _ w386]
              tunnel: w336 -> [w342 w350 w359 w368 w377 _ _]
              frame "Size  **" {
                n201 = Index Array(array=w342) -> (element=w341:cluster{string[]})  [unwired: 1 in]
                n202 = call <vilib>:"NT Read String.vi"("Name"=w344) -> ("String"=w343:string)  [unwired: 9 in, 1 out]
                n203 = property on="Test Slider" class="Slide (strict)"("Visible"=FALSE) -> ()  [unwired: 2 in, 2 out]
                n204 = property on="Test Ring" class="Ring (strict)"("Visible"=TRUE) -> ()  [unwired: 2 in, 2 out]
                n205 = Unbundle(w341) -> (w339:string[])
                n206 = Match First String(2:w339, 3:w343) -> (0:w340:i32)  [unwired: 1 out]
                n207 = property on="Test Ring" class="Ring (strict)"("Value"=w340, "Strings []"=w339) -> ()  [unwired: 2 in, 2 out]
              }
              frame "White Balance  **" {
                n208 = call <vilib>:"NT Read String.vi"("Name"=w353) -> ("String"=w352:string)  [unwired: 9 in, 1 out]
                n209 = Index Array(array=w350, index=1) -> (element=w351:cluster{string[]})
                n210 = property on="Test Slider" class="Slide (strict)"("Visible"=FALSE) -> ()  [unwired: 2 in, 2 out]
                n211 = property on="Test Ring" class="Ring (strict)"("Visible"=TRUE) -> ()  [unwired: 2 in, 2 out]
                n212 = Unbundle(w351) -> (w348:string[])
                n213 = Match First String(2:w348, 3:w352) -> (0:w347:i32)  [unwired: 1 out]
                n214 = property on="Test Ring" class="Ring (strict)"("Value"=w347, "Strings []"=w348) -> ()  [unwired: 2 in, 2 out]
              }
              frame "Exposure  **" {
                n215 = call <vilib>:"NT Read String.vi"("Name"=w362) -> ("String"=w361:string)  [unwired: 9 in, 1 out]
                n216 = Index Array(array=w359, index=2) -> (element=w360:cluster{string[]})
                n217 = property on="Test Slider" class="Slide (strict)"("Visible"=FALSE) -> ()  [unwired: 2 in, 2 out]
                n218 = property on="Test Ring" class="Ring (strict)"("Visible"=TRUE) -> ()  [unwired: 2 in, 2 out]
                n219 = Unbundle(w360) -> (w356:string[])
                n220 = Match First String(2:w356, 3:w361) -> (0:w357:i32)  [unwired: 1 out]
                n221 = property on="Test Ring" class="Ring (strict)"("Value"=w357, "Strings []"=w356) -> ()  [unwired: 2 in, 2 out]
              }
              frame "Exposure Priority  **" {
                n222 = call <vilib>:"NT Read String.vi"("Name"=w371) -> ("String"=w370:string)  [unwired: 9 in, 1 out]
                n223 = Index Array(array=w368, index=3) -> (element=w369:cluster{string[]})
                n224 = property on="Test Slider" class="Slide (strict)"("Visible"=FALSE) -> ()  [unwired: 2 in, 2 out]
                n225 = property on="Test Ring" class="Ring (strict)"("Visible"=TRUE) -> ()  [unwired: 2 in, 2 out]
                n226 = Unbundle(w369) -> (w365:string[])
                n227 = Match First String(2:w365, 3:w370) -> (0:w366:i32)  [unwired: 1 out]
                n228 = property on="Test Ring" class="Ring (strict)"("Value"=w366, "Strings []"=w365) -> ()  [unwired: 2 in, 2 out]
              }
              frame "Color Enable  **" {
                n229 = call <vilib>:"NT Read String.vi"("Name"=w380) -> ("String"=w379:string)  [unwired: 9 in, 1 out]
                n230 = Index Array(array=w377, index=4) -> (element=w378:cluster{string[]})
                n231 = property on="Test Slider" class="Slide (strict)"("Visible"=FALSE) -> ()  [unwired: 2 in, 2 out]
                n232 = property on="Test Ring" class="Ring (strict)"("Visible"=TRUE) -> ()  [unwired: 2 in, 2 out]
                n233 = Unbundle(w378) -> (w374:string[])
                n234 = Match First String(2:w374, 3:w379) -> (0:w375:i32)  [unwired: 1 out]
                n235 = property on="Test Ring" class="Ring (strict)"("Value"=w375, "Strings []"=w374) -> ()  [unwired: 2 in, 2 out]
              }
              frame Default {
                n236 = property on="Test Slider" class="Slide (strict)"("Visible"=FALSE) -> ()  [unwired: 2 in, 2 out]
                n237 = property on="Test Ring" class="Ring (strict)"("Visible"=FALSE) -> ()  [unwired: 2 in, 2 out]
              }
              frame "Brightness  **", "Color Level  **", "Compression  **", "FPS  **", "Sharpness  **" {
                n238 = call <vilib>:"NT Read Number.vi"("Name"=w386) -> ("Numeric"=w385:dbl)  [unwired: 9 in, 1 out]
                n239 = property on="Test Ring" class="Ring (strict)"("Visible"=FALSE) -> ()  [unwired: 2 in, 2 out]
                n240 = property on="Test Slider" class="Slide (strict)"("Visible"=TRUE, "Scale.Maximum"=100.0 ("Scale.Range:Maximum")) -> ()  [unwired: 2 in, 2 out]
                n241 = local write "Test Slider"(w385) -> ()
              }
            }
            n242 = property on="Motor" class="Clust (strict)"("Visible"=FALSE) -> ()  [unwired: 2 in, 2 out]
            n243 = property on="Rev/Fwd" class="Clust (strict)"("Visible"=FALSE) -> ()  [unwired: 2 in, 2 out]
          }
        }
      }
      event "Test Name": Mouse Enter {
        # "Populate the ring with the list of tests"
        n244 = event-data() -> ()  [unwired: 1 in, 1 out]
        n245 = call <vilib>:"NT Read String Array.vi"("Name"="/TestMode/TestList") -> ("String Array"=w394:string[])  [unwired: 9 in, 1 out]
        n246 = Build Array (concatenate)("Select the test to run...", w394) -> (w393:string[])
        n247 = property on="Test Name" class="Ring (strict)"("Strings []"=w393) -> ()  [unwired: 2 in, 2 out]
      }
      event "Test Name": Value Change {
        w396 = FALSE ("Visible")
        # "Tell the robot the test name to run"
        n248 = event-data() -> ("NewVal"=w400:u16)  [unwired: 1 in]
        n249 = property on="Test Name" class="Ring (strict)"() -> ("Strings []"=w401:string[])  [unwired: 2 in, 2 out]
        n250 = local write "Progress"(T6 {"Test Progress"=0, "Test Progress Text"=""} ("Progress")) -> ()
        n251 = property on="Progress" class="Clust (strict)"("Visible"=TRUE) -> ()  [unwired: 2 in, 2 out]
        n252 = property on="Test Ring" class="Ring (strict)"("Visible"=w396) -> ()  [unwired: 2 in, 2 out]
        n253 = property on="Motor" class="Clust (strict)"("Visible"=w396) -> ()  [unwired: 2 in, 2 out]
        n254 = property on="Test Slider" class="Slide (strict)"("Visible"=w396) -> ()  [unwired: 2 in, 2 out]
        n255 = property on="On/Off" class="Bool (strict)"("Visible"=w396) -> ()  [unwired: 2 in, 2 out]
        n256 = property on="Rev/Fwd" class="Clust (strict)"("Visible"=w396) -> ()  [unwired: 2 in, 2 out]
        n257 = Index Array(array=w401, index=w400) -> (element=w399:string)
        n258 = call <vilib>:"NT Write String.vi"("String"=w399, "Name"="/TestMode/TestName") -> ()  [unwired: 9 in, 1 out]
      }
      event "Select Auto": Mouse Enter {
        # "Populate the combo box with the list of autonomous options"
        n259 = event-data() -> ()  [unwired: 1 in, 1 out]
        n260 = call <vilib>:"NT Read String Array.vi"("Name"="Auto List") -> ("String Array"=w403:string[])  [unwired: 9 in, 1 out]
        n261 = property on="Select Auto" class="CmbBox"("Strings[]"=w403) -> ()  [unwired: 2 in, 2 out]
      }
      event "Select Auto": Value Change {
        # "User modified the Auto Selection. Write to NT variable so robot knows."
        n262 = event-data() -> ("NewVal"=w406:string)  [unwired: 1 in]
        n263 = call <vilib>:"NT Write String.vi"("String"=w406, "Name"="Auto Selector") -> ()  [unwired: 9 in, 1 out]
      }
      event "Command Selection": Value Change {
        # "Get the params and show in table"
        n264 = event-data() -> ("NewVal"=w412:i32)  [unwired: 1 in]
        n265 = property on="Command Selection" class="MCListbox (strict)"() -> ("ItemNames"=w410:string[][])  [unwired: 2 in, 2 out]
        n266 = call <vilib>:"WPI_DashboardUpdate Command Params.vi"("NewVal"=w412, "Commands"=w410, "Param Tbl"=w411) -> ()  [unwired: 8 in, 1 out]
      }
      event "Execute Command": Value Change {
        # "Started one, Unique ID holds\nresponse"
        n267 = event-data() -> ()  [unwired: 1 in, 1 out]
        n268 = property on="Command Selection" class="MCListbox (strict)"() -> ("ItemNames"=w423:string[][])  [unwired: 2 in, 2 out]
        n269 = Index Array(array=w423, index (row)="Command Selection", index (col)=0) -> (element=w421:string)
        n270 = call <vilib>:"Invoke Commands.vi"("Command Params"="Command Params", "Function Name"=w421) -> ("Params"=w417:u8, "Started"=w416:bool)  [unwired: 7 in, 1 out]
        n271 = Array Subset(array="Command Params", length (row)=w417) -> (w418:string[][])  [unwired: 3 in]
        n272 = Select(t="Executing" ("Cmd Status"), s=w416, f="" ("Cmd Status")) -> (s? t:f=→"Cmd Status":string)
      }
      event "Command Selection": Double Click {
        n273 = event-data() -> ("Row"=w431:i32)  [unwired: 1 in]
        n274 = property on="Command Selection" class="MCListbox (strict)"() -> ("ItemNames"=w434:string[][])  [unwired: 2 in, 2 out]
        n275 = local read "Command Params"() -> (w430:string[][])
        n276 = Index Array(array=w434, index (row)=w431, index (col)=0) -> (element=w432:string)
        n277 = call <vilib>:"Invoke Commands.vi"("Command Params"=w430, "Function Name"=w432) -> ("Params"=w429:u8, "Started"=w424:bool)  [unwired: 7 in, 1 out]
        n278 = Array Subset(array=w430, length (row)=w429) -> (w428:string[][])  [unwired: 3 in]
        n279 = Select(t="Executing" ("Cmd Status"), s=w424, f="" ("Cmd Status")) -> (s? t:f=w425:string)
        n280 = local write "Cmd Status"(w425) -> ()
      }
      event "CheckList": Double Click {
        # "Shift clears all"
        # "Update symbols on the listbox"
        n281 = event-data() -> ("PlatMods.Shift"=w436:bool, "Row"=w438:i32)  [unwired: 1 in]
        n282 = case shown="True" w436 {
          tunnel: w438 -> [w442 _]
          tunnel: 1 -> [w441 _]
          frame False {
            n283 = property on="CheckList" class="LstBox (strict)"() -> ("Item Symbols"=w440:i32[])  [unwired: 2 in, 2 out]
            n284 = Replace Array Subset(array=w440, new element=w441, index=w442) -> (w439:i32[])
            n285 = property on="CheckList" class="LstBox (strict)"("Item Symbols"=w439) -> ()  [unwired: 2 in, 2 out]
          }
          frame True {
            w443 = 0 ("Top Row")
            n286 = property on="CheckList" class="LstBox (strict)"() -> ("Number of Rows"=w445:u32)  [unwired: 2 in, 2 out]
            n287 = Initialize Array(0, w445) -> (w444:i32[])
            n288 = property on="CheckList" class="LstBox (strict)"("Top Row"=w443, "Value"=w443, "Item Symbols"=w444) -> ()  [unwired: 2 in, 2 out]
          }
        }
      }
      event "CheckList": Key Down {
        # "Update symbols on the listbox\nLeft and right keys check and uncheck"
        n289 = event-data() -> ("VKey"=w449:T19)  [unwired: 1 in]
        n290 = case shown="\"Left\", \"Right\"" w449 {
          selector: w449 -> [w454 _]
          tunnel: eventvkey."Left" ("VKey") -> [w452 _]
          frame "Left", "Right" {
            n291 = Equal?(x=w452, y=w454) -> (x = y?=w453:bool)
            n292 = Select(t=0, s=w453, f=1) -> (s? t:f=w455:i32)
            n293 = property on="CheckList" class="LstBox (strict)"() -> ("Item Symbols"=w458:i32[])  [unwired: 2 in, 2 out]
            n294 = Replace Array Subset(array=w458, new element=w455, index="CheckList") -> (w457:i32[])
            n295 = property on="CheckList" class="LstBox (strict)"("Item Symbols"=w457) -> ()  [unwired: 2 in, 2 out]
          }
          frame Default {
          }
        }
      }
      event "Motor.Enable": Value Change {
        # "When the test mode otor enable helper is set, update that\ntree row item's value"
        n296 = event-data() -> ("NewVal"=w464:bool)  [unwired: 1 in]
        n297 = Unbundle("Motor") -> ("Value"=w463:dbl)  [unwired: 1 out]
        n298 = Select(t=w463, s=w464, f=0.0) -> (s? t:f=w461:dbl)
        n299 = call <vilib>:"NT Write Number.vi"("Numeric"=w461, "Name"=w460) -> ()  [unwired: 9 in, 1 out]
      }
      event "Test Slider": Value Change {
        # "When the test mode slider helper is set, update that\ntree row item's value"
        n300 = event-data() -> ("NewVal"=w467:dbl)  [unwired: 1 in]
        n301 = call <vilib>:"NT Write Number.vi"("Numeric"=w467, "Name"=w468) -> ()  [unwired: 9 in, 1 out]
      }
      event "On/Off": Value Change {
        # "When the test mode on/off helper value is set, update that\ntree row item's value"
        n302 = event-data() -> ("NewVal"=w472:bool)  [unwired: 1 in]
        n303 = Boolean To (0,1)(Boolean=w472) -> (0, 1=w471:i16)
        n304 = call <vilib>:"NT Write Number.vi"("Numeric"=w471, "Name"=w470) -> ()  [unwired: 9 in, 1 out]
      }
      event "Rev/Fwd": Value Change {
        # "When the test mode helper value for relays is set, update that\ntree row item's value"
        n305 = event-data() -> ("NewVal.Forward"=w480:bool, "NewVal.Reverse"=w479:bool)  [unwired: 1 in]
        n306 = Boolean To (0,1)(Boolean=w480) -> (0, 1=w476:i16)
        n307 = Boolean To (0,1)(Boolean=w479) -> (0, 1=w478:i16)
        n308 = Negate(x=w478) -> (-x=w477:i16)
        n309 = Add(x=w476, y=w477) -> (x+y=w475:i16)
        n310 = call <vilib>:"NT Write Number.vi"("Numeric"=w475, "Name"=w474) -> ()  [unwired: 9 in, 1 out]
      }
      event "Test Ring": Value Change {
        # "When a test mode helper value is selected from the ring,\nset the tree item's variable to the string value"
        n311 = event-data() -> ("NewVal"=w484:u16)  [unwired: 1 in]
        n312 = property on="Test Ring" class="Ring (strict)"() -> ("Strings []"=w485:string[])  [unwired: 2 in, 2 out]
        n313 = Index Array(array=w485, index=w484) -> (element=w483:string)
        n314 = call <vilib>:"NT Write String.vi"("String"=w483, "Name"=w482) -> ()  [unwired: 9 in, 1 out]
      }
      event "Rec Mode": Value Change {
        # "Update globals for recording mode and path to read log from.\nClear when logging and let NetworkTables set path for vision to\nuse."
        n315 = event-data() -> ("NewVal"=w496:enum32{"Stop", "Record", "Playback"})  [unwired: 1 in]
        n316 = global write "WPI_DashboardLogging Global.vi" "Recording"(w496) -> ()
        n317 = global write "WPI_DashboardLogging Global.vi" "Logging Filename"(path "") -> ()
        n318 = case shown="\"Playback\"" w496 {
          tunnel: w495 -> [_ w498 w507]
          tunnel: [_ _ w506] -> w493
          tunnel: [_ _ w505] -> _
          tunnel: w491 -> [_ _ w503]
          tunnel: cluster{i32, i32} {-250, 170} -> [_ _ w502]
          tunnel: [_ _ T20 {"Image Size"=TRUE, "Image Type"=TRUE, "Pixel Value"=TRUE, "ROI Information"=TRUE, "Zoom Factor"=FALSE} ("Image Information Shown:All Elements")] -> w489
          tunnel: [_ _ TRUE ("Zoom Factor")] -> w488
          tunnel: w487 -> [_ _ w499]
          frame Default {
          }
          frame "Stop", "Record" {
            # "Place Window too"
            n319 = invoke class="VI" method="FP.Close"(reference=w498) -> (reference out=w497:refnum<vi>)  [unwired: 2 in, 2 out]
            n320 = invoke class="VI" method="Abort VI"(reference=w497) -> ()  [unwired: 2 in, 3 out]
          }
          frame "Playback" {
            n321 = call "Open Playback Panel.vi"("Offset"=w502, "DB VI Ref"=w503, "Playback in"=w507) -> ("Playback out"=w504:refnum<vi>)  [unwired: 8 in]
            n322 = register-events(w504, w499) -> (reference out=w506:refnum<event-registration>, error out=w505:errorcluster)  [unwired: 2 in]
          }
        }
        n323 = call <vilib>:"WPI_DashboardNT Log FieldName Cache.vi"("Operation"=enum16{"Lookup/Add", "Index", "Clear"}."Clear") -> ()  [unwired: 8 in, 3 out]
        n324 = property on="Camera Image" class="ImageControl"("Image Information Shown"=w489, "Image Information Visible"=w488) -> ()  [unwired: 2 in, 2 out]
      }
      event Panel Close {
        w509 = enum32{"Stop", "Record", "Playback"}."Stop" ("Rec Mode")
        # "Playback window has been closed, abort"
        n325 = event-data() -> ()  [unwired: 1 in, 4 out]
        n326 = local write "Rec Mode"(w509) -> ()
        n327 = global write "WPI_DashboardLogging Global.vi" "Recording"(w509) -> ()
      }
      event Panel Close {
        # "Abort playback window and ourself"
        n328 = event-data() -> ()  [unwired: 1 in, 4 out]
        n329 = invoke class="VI" method="FP.Close"(reference=w513) -> (reference out=w512:refnum<vi>)  [unwired: 2 in, 2 out]
        n330 = invoke class="VI" method="Abort VI"(reference=w512) -> (error out=w511:errorcluster)  [unwired: 2 in, 2 out]
        n331 = invoke class="VI" method="Abort VI"(error in=w511) -> ()  [unwired: 2 in, 3 out]
      }
      event User Event {
        n332 = event-data() -> ("IDs"=w520:cluster{"RPC field ID":u16, "Unique ID":u16}, "String"=w519:string)  [unwired: 1 in]
        n333 = Bundle("IDs"=w520, "String"=w519) -> (w518:T8)  [unwired: 1 in]
        n334 = local write "Cmd Status"("" ("Cmd Status")) -> ()
        n335 = call <vilib>:"Retrieve RPC Response.vi"("RPC Response"=w518) -> ("Output"=w516:string[][])  [unwired: 10 in]
        n336 = Build Array (concatenate)(w514, w516) -> (w515:string[][])
        n337 = local write "Command Params"(w515) -> ()
      }
      event "Tree": Double Click {
        n338 = event-data() -> ("PlatMods"=w524:T23, "Tag"=w523:string)  [unwired: 1 in]
        n339 = Unbundle(w524) -> ("Shift"=w522:bool)  [unwired: 4 out]
        n340 = Not(x=w522) -> (.not. x?=w521:bool)
        n341 = call <vilib>:"NT Update Persistence.vi"("Persistence"=w521, "Name"=w523) -> ()  [unwired: 9 in, 1 out]
      }
    }
  }
  n342 = while {
    tunnel: w57 -> [w537]
    tunnel: w35 -> [w535]
    tunnel: [w533] -> _
    tunnel: u32 1000 ("milliseconds to wait") -> [w532]
    tunnel: w25 -> [w526]
    i -> [w533]
    stop <- FALSE stop-if-true
    n343 = Wait on Notification(notifier=w535, timeout in ms (-1)=w532) -> (notification=w534:string, timed out?=w530:bool)  [unwired: 2 in, 2 out]
    n344 = local read "Rec Mode"() -> (w528:enum32{"Stop", "Record", "Playback"})
    n345 = Equal?(x=w528, y=u16 2 ("Rec Mode")) -> (x = y?=w529:bool)
    n346 = Compound Arithmetic op=OR(invert w530, w529) -> (w531:bool)
    n347 = case shown="True" w531 {
      tunnel: w537 -> [_ w540]
      tunnel: w534 -> [_ w539]
      tunnel: w526 -> [_ w538]
      frame False {
      }
      frame True {
        n348 = call <vilib>:"Bind Controls to SmartDashboard.vi"("RPC ref"=w538, "Bound Control Refs"=w540, "Server IP Address"=w539) -> ()  [unwired: 9 in]
      }
    }
  }
